vi "Get ring selector channels and groups .vi"(10 "Plots  selector":cluster{"X":u16, "Y":u16}[](array[cluster]) {"Y" items=["Select channel...", "Time", "Y"]; "X" items=["Select channel...", "Time", "Y"]}, 11 "File-group-channel":T1(array[cluster])) -> (0 "Channels Y":string[](array[string]), 1 "Groups Y":string[](array[string]), 2 "Channels X":string[](array[string]), 3 "Groups X":string[](array[string]))   [LabVIEW 2019]
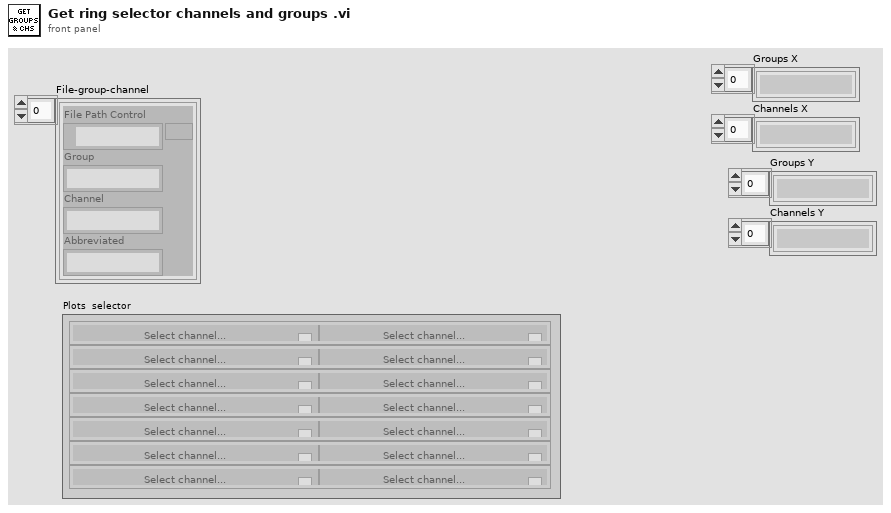
[diagram p1: front panel]
types:
  T1 = cluster{"File Path Control":path, "Group":string, "Channel":string, "Abbreviated":string}[]
  T2 = cluster{"File Path Control":path, "Group":string, "Channel":string, "Abbreviated":string}
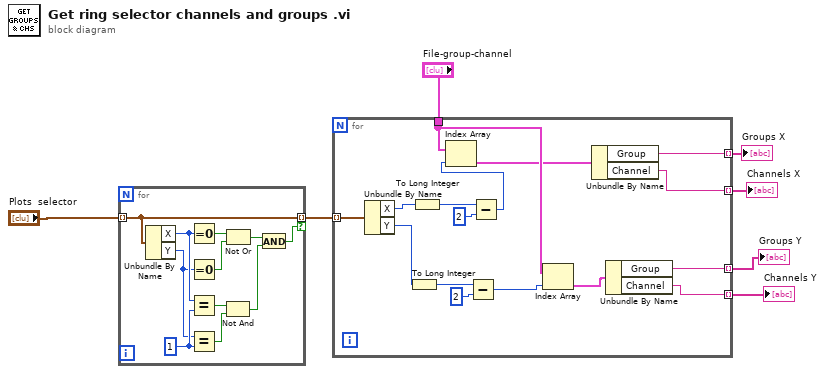
[diagram p0: block diagram]
diagram:
  n1 = for {
    tunnel: "Plots  selector" -> [w16] mode=indexing
    tunnel: [w16] -> w6 mode=indexing if=w9
    w13 = u16 1 ("y")
    n2 = Unbundle By Name(w16) -> ("X"=w14:u16, "Y"=w12:u16)
    n3 = Equal To 0?(x=w14) -> (x = 0?=w18:bool)
    n4 = Equal To 0?(x=w12) -> (x = 0?=w17:bool)
    n5 = Equal?(x=w14, y=w13) -> (x = y?=w11:bool)
    n6 = Equal?(x=w12, y=w13) -> (x = y?=w10:bool)
    n7 = Not Or(1:w17, 2:w18) -> (0:w15:bool)
    n8 = Not And(1:w10, 2:w11) -> (0:w8:bool)
    n9 = And(x=w15, y=w8) -> (x .and. y?=w9:bool)
  }
  n10 = for {
    tunnel: w6 -> [w34] mode=indexing
    tunnel: "File-group-channel" -> [w26]
    tunnel: [w22] -> w4 mode=indexing
    tunnel: [w21] -> w3 mode=indexing
    tunnel: [w20] -> w2 mode=indexing
    tunnel: [w19] -> w1 mode=indexing
    n11 = Unbundle By Name(w34) -> ("X"=w29:u16, "Y"=w28:u16)
    n12 = To Long Integer(number=w28) -> (32bit integer=w31:i32)
    n13 = To Long Integer(number=w29) -> (32bit integer=w33:i32)
    n14 = Subtract(x=w31, y=2) -> (x-y=w25:i32)
    n15 = Subtract(x=w33, y=2) -> (x-y=w27:i32)
    n16 = Index Array(array=w26, index=w27) -> (element=w24:T2)
    n17 = Index Array(array=w26, index=w25) -> (element=w23:T2)
    n18 = Unbundle By Name(w24) -> ("Group"=w22:string, "Channel"=w21:string)
    n19 = Unbundle By Name(w23) -> ("Group"=w20:string, "Channel"=w19:string)
  }
  "Groups X" <- w4
  "Channels X" <- w3
  "Groups Y" <- w2
  "Channels Y" <- w1
